vi "To U64.vi"   [LabVIEW 2017]
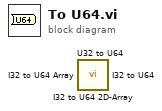
[diagram p0: block diagram]
diagram:
  n1 = call <vilib>:"I32 to U64 2D-Array.vi"() -> ()  [unwired: 1 in, 1 out]
  n2 = call <vilib>:"U32 to U64.vi"() -> ()  [unwired: 1 in, 1 out]
  n3 = call <vilib>:"I32 to U64 Array.vi"() -> ()  [unwired: 1 in, 1 out]
  n4 = call <vilib>:"I32 to U64.vi"() -> ()  [unwired: 1 in, 1 out]
